vi "Error_and_Status.vi"(8 "error in (no error)":errorcluster, 9 "Retry interval (ms)":u32, 10 "Number of tries":u32, 11 "ES Packet":T2) -> (0 "error out":errorcluster, 2 "ES Param Out":T1, 3 "ES Packet Out":T2)   [LabVIEW 2017]
uses:
  Controls/Packet/Packet.ctl
  Controls/Packet/Packet_Direction.ctl
  Controls/Packet/Packet_Type.ctl
  Controls/Packet/Packet_Priority.ctl
  Controls/Control Packets/ES_Param.ctl
  <vilib>/Instr/_visa.llb/VISA Flush IO Buffer Mask.ctl
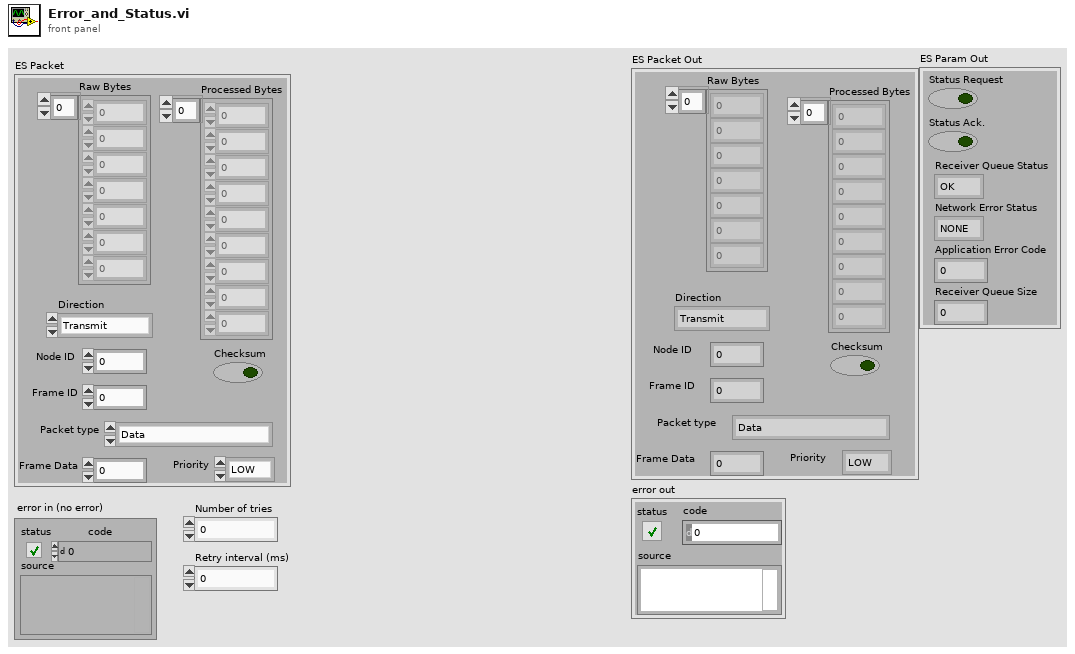
[diagram p1: front panel]
types:
  T1 = typedef "ES_Param.ctl" = cluster{"Status Request":bool, "Status Ack.":bool, "Receiver Queue Status":enum16{"OK", "EMPTY", "FULL"}, "Network Error Status":enum16{"NONE", "CONNECTION_ALREADY_OPEN", "CONNECTION_ALREADY_CLOSED", "INVALID_FRAME_REQUEST"}, "Application Error Code":u16, "Receiver Queue Size":i32}
  T2 = typedef "Packet.ctl" = cluster{"Raw Bytes":u8[], "Checksum":bool, "Direction":T3, "Processed Bytes":u8[], "Node ID":u8, "Packet type":T4, "Frame Data":u32, "Priority":T5, "Frame ID":u8}
  T3 = typedef "Packet_Direction.ctl" = enum16{"Transmit", "Receive", "Bidirectional"}
  T4 = typedef "Packet_Type.ctl" = enum16{"Data", "Connection Management", "Remote Request", "Error/Status"}
  T5 = typedef "Packet_Priority.ctl" = enum16{"LOW", "HIGH"}
  T6 = typedef "VISA Flush IO Buffer Mask.ctl" = u16
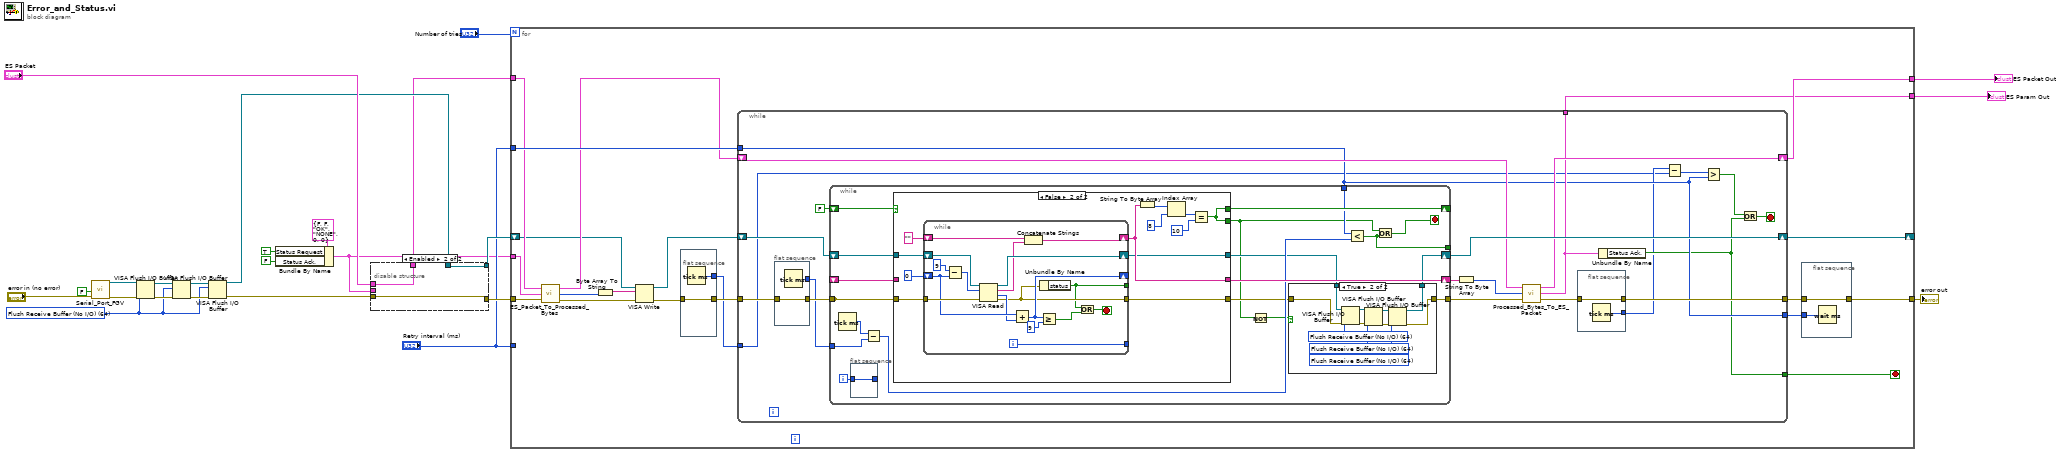
[diagram p0: block diagram]
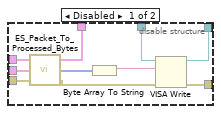
[diagram p2: hidden frame]
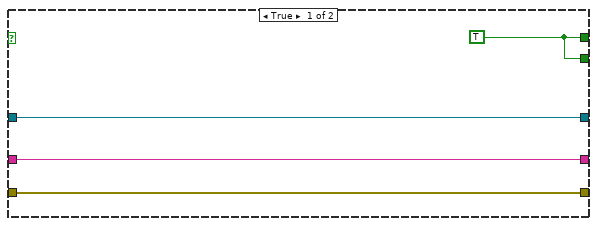
[diagram p4: hidden frame]
diagram:
  w16 = T6 64 items=["Flush Receive Buffer"=16, "Write Transmit Buffer to Device"=32, "Flush Receive Buffer (No I/O)"=64, "Flush Transmit Buffer"=128] ("Mask")
  n1 = call "Serial_Port_FGV.vi"("error in (no error)"="error in (no error)", "Initialize ?"=FALSE) -> ("error out"=w22:errorcluster, "COM Port out"=w21:refnum<visa-resource-name>)  [unwired: 8 in]
  n2 = VISA Flush I/O Buffer(VISA resource name=w21, mask (16)=w16, error in (no error)=w22) -> (VISA resource name out=w20:refnum<visa-resource-name>, error out=w19:errorcluster)
  n3 = VISA Flush I/O Buffer(VISA resource name=w20, mask (16)=w16, error in (no error)=w19) -> (VISA resource name out=w18:refnum<visa-resource-name>, error out=w17:errorcluster)
  n4 = VISA Flush I/O Buffer(VISA resource name=w18, mask (16)=w16, error in (no error)=w17) -> (VISA resource name out=w10:refnum<visa-resource-name>, error out=w12:errorcluster)
  n5 = Bundle By Name(cluster=T1 {"Status Request"=FALSE, "Status Ack."=FALSE, "Receiver Queue Status"=enum."OK", "Network Error Status"=enum."NONE", "Application Error Code"=0, "Receiver Queue Size"=0} ("Cluster"), "Status Request"=TRUE, "Status Ack."=FALSE) -> (w1:T1)
  n6 = disable-structure shown="Enabled" {
    disable-tunnel: w12 -> [w34 w35]
    disable-tunnel: "ES Packet" -> [w33 w36]
    disable-tunnel: w10 -> [w30 w37]
    disable-tunnel: [w28 w35] -> w9
    disable-tunnel: [w27 w37] -> w8
    disable-tunnel: [w26 w36] -> w5
    disable-tunnel: w1 -> [w25 _]
    frame Disabled {
      n7 = call "ES_Packet_To_Processed_Bytes.vi"("error in (no error)"=w34, "ES Param In"=w25, "ES Packet In"=w33) -> ("error out"=w31:errorcluster, "Processed Bytes"=w32:u8[], "ES Packet Out"=w26:T2)
      n8 = Byte Array To String(unsigned byte array=w32) -> (string=w29:string)
      n9 = VISA Write(VISA resource name=w30, write buffer=w29, error in (no error)=w31) -> (VISA resource name out=w27:refnum<visa-resource-name>, error out=w28:errorcluster)  [unwired: 1 out]
    }
    frame Enabled {
    }
  }
  n10 = for {
    N: "Number of tries" -> [_]
    tunnel: w9 -> [w48]
    shift-right: [w56] -> _
    shift-left: w8 -> [w40]
    tunnel: "Retry interval (ms)" -> [_]
    tunnel: "Retry interval (ms)" -> [w57]
    tunnel: w5 -> [w47]
    tunnel: [w55] -> w4
    tunnel: [w54] -> w3
    tunnel: [w52] -> w2
    tunnel: w1 -> [w45]
    stop <- w49 stop-if-true
    n11 = call "ES_Packet_To_Processed_Bytes.vi"("error in (no error)"=w48, "ES Param In"=w45, "ES Packet In"=w47) -> ("error out"=w43:errorcluster, "Processed Bytes"=w42:u8[], "ES Packet Out"=w46:T2)
    n12 = Byte Array To String(unsigned byte array=w42) -> (string=w44:string)
    n13 = VISA Write(VISA resource name=w40, write buffer=w44, error in (no error)=w43) -> (VISA resource name out=w39:refnum<visa-resource-name>, error out=w41:errorcluster)  [unwired: 1 out]
    n14 = flat-sequence {
      tunnel: w41 -> [w59]
      tunnel: [w59] -> w50
      tunnel: [w58] -> w38
      frame #0 {
        n15 = Tick Count (ms)() -> (millisecond timer value=w58:u32)
      }
    }
    n16 = while {
      tunnel: w50 -> [w74]
      tunnel: w38 -> [w63]
      tunnel: w57 -> [w69]
      tunnel: [w75] -> w54
      shift-right: [w81] -> w56
      shift-left: w39 -> [w82]
      shift-right: [w76] -> w55
      shift-left: w46 -> [w79]
      tunnel: [w70] -> w53
      tunnel: [w69] -> w51
      tunnel: [w68] -> w49
      stop <- w71 stop-if-true
      n17 = flat-sequence {
        tunnel: w74 -> [w86]
        tunnel: [w86] -> w73
        tunnel: [w85] -> w64
        frame #0 {
          n18 = Tick Count (ms)() -> (millisecond timer value=w85:u32)
        }
      }
      n19 = while {
        tunnel: w73 -> [w100]
        shift-right: [w103] -> _
        shift-left: FALSE -> [w104]
        tunnel: [w94] -> w80
        shift-right: [w102] -> w78
        shift-left: _ -> [w101]
        shift-right: [w92] -> w81
        shift-left: w82 -> [w105]
        tunnel: [w100] -> _
        tunnel: w64 -> [w98]
        tunnel: w69 -> [w96]
        tunnel: [w87] -> _
        i -> [w91]
        stop <- w90 stop-if-true
        n20 = Tick Count (ms)() -> (millisecond timer value=w99:u32)
        n21 = flat-sequence {
          tunnel: w91 -> [w106]
          tunnel: [w106] -> _
          frame #0 {
          }
        }
        n22 = Subtract(x=w99, y=w98) -> (x-y=w97:u32)
        n23 = case shown="False" w104 {
          tunnel: w100 -> [w122 w135]
          tunnel: w105 -> [w120 w133]
          tunnel: [w123 w127] -> w88
          tunnel: [w123 w127] -> w103
          tunnel: [w122 w126] -> w95
          tunnel: [w121 w125] -> w102
          tunnel: w101 -> [w121 _]
          tunnel: [w120 w124] -> w93
          frame True {
            w123 = TRUE
          }
          frame False {
            n24 = while {
              tunnel: w135 -> [w152]
              shift-right: [w142] -> _
              shift-left: 0 -> [w145]
              shift-right: [w148] -> w124
              shift-left: w133 -> [w149]
              shift-right: [w141] -> w125
              shift-left: "" -> [w147]
              tunnel: [w139] -> w126
              tunnel: [w140] -> _
              tunnel: [w136] -> _
              i -> [w140]
              stop <- w138 stop-if-true
              n25 = Subtract(x=9, y=w145) -> (x-y=w150:u32)
              n26 = VISA Read(VISA resource name=w149, byte count=w150, error in (no error)=w152) -> (VISA resource name out=w148:refnum<visa-resource-name>, read buffer=w146:string, return count=w144:u32, error out=w139:errorcluster)
              n27 = Add(x=w145, y=w144) -> (x+y=w142:u32)
              n28 = Concatenate Strings(w147, w146) -> (w141:string)
              n29 = Unbundle By Name(w139) -> ("status"=w136:bool)
              n30 = Greater Or Equal?(x=w142, y=u32 9) -> (x >= y?=w137:bool)
              n31 = Or(x=w136, y=w137) -> (x .or. y?=w138:bool)
            }
            n32 = String To Byte Array(string=w125) -> (unsigned byte array=w131:u8[])
            n33 = Index Array(array=w131, index=8) -> (element=w129:u8)
            n34 = Equal?(x=w129, y=u8 10) -> (x = y?=w127:bool)
          }
        }
        n35 = Not(x=w88) -> (.not. x?=w89:bool)
        n36 = case shown="True" w89 {
          tunnel: w95 -> [w108 w119]
          tunnel: [w108 w116] -> w94
          tunnel: w93 -> [w107 w115]
          tunnel: [w107 w112] -> w92
          frame False {
          }
          frame True {
            w109 = T6 64 items=["Flush Receive Buffer"=16, "Write Transmit Buffer to Device"=32, "Flush Receive Buffer (No I/O)"=64, "Flush Transmit Buffer"=128] ("Mask")
            w110 = T6 64 items=["Flush Receive Buffer"=16, "Write Transmit Buffer to Device"=32, "Flush Receive Buffer (No I/O)"=64, "Flush Transmit Buffer"=128] ("Mask")
            w111 = T6 64 items=["Flush Receive Buffer"=16, "Write Transmit Buffer to Device"=32, "Flush Receive Buffer (No I/O)"=64, "Flush Transmit Buffer"=128] ("Mask")
            n37 = VISA Flush I/O Buffer(VISA resource name=w115, mask (16)=w111, error in (no error)=w119) -> (VISA resource name out=w114:refnum<visa-resource-name>, error out=w118:errorcluster)
            n38 = VISA Flush I/O Buffer(VISA resource name=w114, mask (16)=w110, error in (no error)=w118) -> (VISA resource name out=w113:refnum<visa-resource-name>, error out=w117:errorcluster)
            n39 = VISA Flush I/O Buffer(VISA resource name=w113, mask (16)=w109, error in (no error)=w117) -> (VISA resource name out=w112:refnum<visa-resource-name>, error out=w116:errorcluster)
          }
        }
        n40 = Less?(x=w96, y=w97) -> (x < y?=w87:bool)
        n41 = Or(x=w88, y=w87) -> (x .or. y?=w90:bool)
      }
      n42 = String To Byte Array(string=w78) -> (unsigned byte array=w77:u8[])
      n43 = call "Processed_Bytes_To_ES_Packet.vi"("error in (no error)"=w80, "Processed_Bytes"=w77, "ES Packet In"=w79) -> ("error out"=w72:errorcluster, "ES Param Out"=w75:T1, "ES Packet Out"=w76:T2)
      n44 = flat-sequence {
        tunnel: w72 -> [w84]
        tunnel: [w84] -> w70
        tunnel: [w83] -> w66
        frame #0 {
          n45 = Tick Count (ms)() -> (millisecond timer value=w83:u32)
        }
      }
      n46 = Unbundle By Name(w75) -> ("Status Ack."=w68:bool)
      n47 = Subtract(x=w66, y=w63) -> (x-y=w65:u32)
      n48 = Greater?(x=w65, y=w69) -> (0:w62:bool)
      n49 = Or(x=w62, y=w68) -> (x .or. y?=w71:bool)
    }
    n50 = flat-sequence {
      tunnel: w53 -> [w61]
      tunnel: [w61] -> w52
      tunnel: w51 -> [w60]
      frame #0 {
        n51 = Wait (ms)(milliseconds to wait=w60) -> ()  [unwired: 1 out]
      }
    }
  }
  "ES Packet Out" <- w4
  "ES Param Out" <- w3
  "error out" <- w2
